vi "Replace LVClass Name.vi"(7 "Test Case class name":string, 11 "Name in":string) -> (3 "Name out":string)   [LabVIEW 2020, in "Test Finder.lvclass"]
uses:
  Test Finder.lvclass
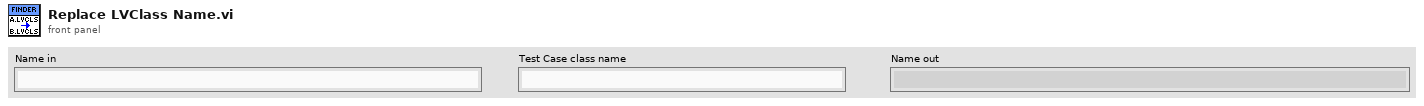
[diagram p1: front panel]
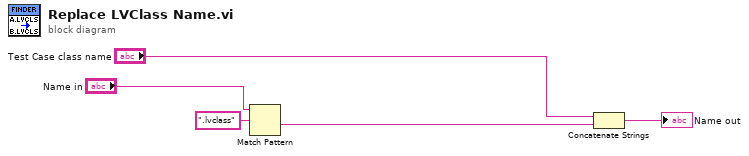
[diagram p0: block diagram]
diagram:
  n1 = Match Pattern(string="Name in", regular expression=".lvclass") -> (after substring=w3:string)  [unwired: 1 in, 3 out]
  n2 = Concatenate Strings("Test Case class name", w3) -> (→"Name out":string)
